vi "Head_Servo_Write.vi"(10 "Stop":bool, 11 "Calibrated Oculus Data":T1) -> ()   [LabVIEW 2017]
uses:
  Calibrated Oculus Data.ctl
  <vilib>/myRIO/Instrument Drivers/Onboard IO/PWM/typedefs/PWM Reference.ctl
  <vilib>/myRIO/Common/Instrument Driver Framework/Utilities/typedefs/myRIO Generic Hardware Reference.ctl
  <vilib>/myRIO/Common/Instrument Driver Framework/Utilities/typedefs/Hardware Version Enum.ctl
  <vilib>/myRIO/Common/Instrument Driver Framework/Utilities/typedefs/myRIO v1.0 Reference.ctl
  <vilib>/myRIO/Common/Instrument Driver Framework/Utilities/typedefs/Generic FPGA Reference.ctl
  <vilib>/myRIO/Common/Instrument Driver Framework/myRIO v1.0/PWM/typedefs/PWM Channels Enum.ctl
  <vilib>/myRIO/Instrument Drivers/Onboard IO/PWM/typedefs/PWM Configuration.ctl
  <vilib>/userdefined/High Color/nirio_resource_hc.ctl
  <vilib>/myRIO/Common/Instrument Driver Framework/Utilities/vis/Is FPGA Ref Available.vi
  <vilib>/myRIO/Common/Instrument Driver Framework/myRIO v1.0/PWM/vis/myRIO v1.1 Open PWM.vi
  <vilib>/myRIO/Instrument Drivers/Onboard IO/PWM/vis/Set Duty Cycle and Frequency.vi
  <vilib>/myRIO/Common/Instrument Driver Framework/Utilities/vis/Validate Channels.vi
  <vilib>/myRIO/Common/Instrument Driver Framework/myRIO v1.0/PWM/vis/myRIO v1.0 Reserve PWM.vi
  <vilib>/myRIO/Common/Instrument Driver Framework/myRIO v1.0/PWM/vis/myRIO v1.0 Build MUX Configuration PWM.vi
  <vilib>/myRIO/Common/Instrument Driver Framework/myRIO v1.0/Resource Manager/vis/myRIO v1.0 Reserve Channel List.vi
  <vilib>/myRIO/Common/Instrument Driver Framework/myRIO v1.0/Resource Manager/vis/myRIO v1.0 Create Configuration List.vi
  <vilib>/myRIO/Common/Instrument Driver Framework/myRIO v1.0/Resource Manager/vis/myRIO v1.0 Reserve Channel.vi
  <vilib>/myRIO/Common/Instrument Driver Framework/myRIO v1.0/Resource Manager/vis/myRIO v1.0 Unreserve Channel.vi
  <vilib>/myRIO/Common/Instrument Driver Framework/myRIO v1.0/Resource Manager/vis/myRIO v1.0 Build Mutex Name.vi
  <vilib>/Utility/VariantDataType/GetNumericInfo.vi
  <vilib>/Utility/error.llb/Error Cluster From Error Code.vi
  <vilib>/myRIO/Common/Instrument Driver Framework/myRIO v1.0/myRIO v1.1 Open.vi
  <vilib>/myRIO/Common/Instrument Driver Framework/Utilities/vis/IO Manager.vi
  <vilib>/myRIO/Common/Instrument Driver Framework/Utilities/vis/Configuration Manager.vi
  <vilib>/myRIO/Common/Instrument Driver Framework/myRIO v1.0/Resource Manager/vis/myRIO v1.0 Configure IO.vi
  <vilib>/myRIO/Common/Instrument Driver Framework/myRIO v1.0/myRIO v1.0 Close.vi
  <vilib>/myRIO/Common/Instrument Driver Framework/myRIO v1.0/PWM/vis/myRIO v1.0 Write PWM.vi
  <vilib>/express/express arith-compare/Formula/XNode/ExpressFormulaBlockNode.xnode
  <vilib>/myRIO/Express VI/Onboard IO/PWM/PWM Express VI.xnode
  <vilib>/myRIO/Instrument Drivers/Onboard IO/PWM/vis/myRIO PWM Open.xnode
  <vilib>/myRIO/Instrument Drivers/Onboard IO/PWM/PWM.lvlib
panel:
  in  "error in":errorcluster
  out "error out":errorcluster
  in  "Pich Offset":dbl
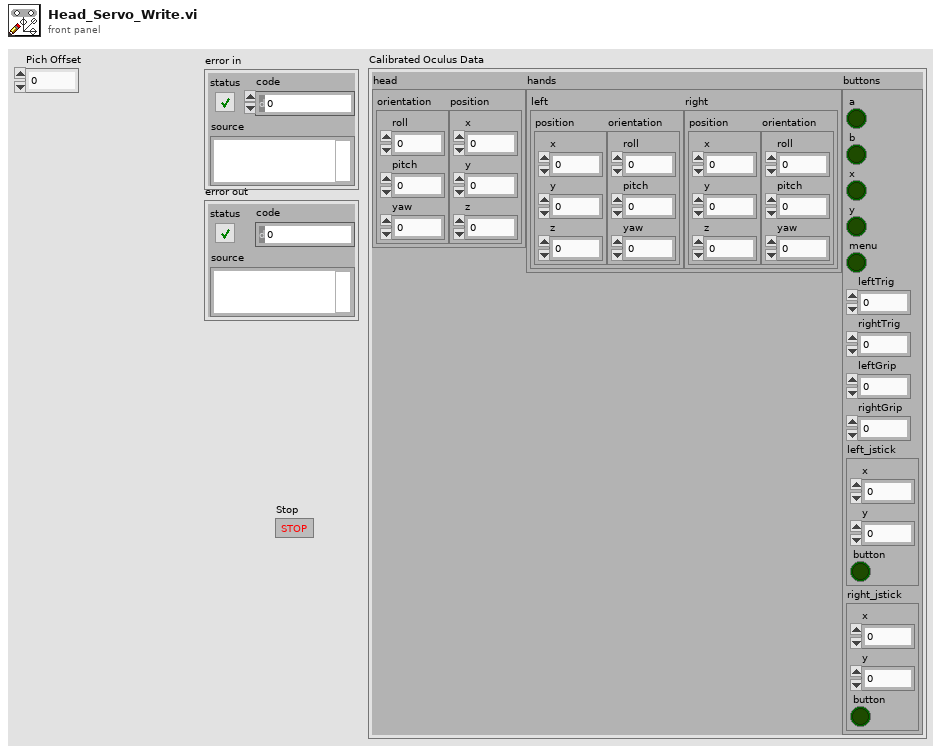
[diagram p1: front panel]
types:
  T1 = typedef "Calibrated Oculus Data.ctl" = cluster{"head":cluster{"orientation":cluster{"roll":dbl, "pitch":dbl, "yaw":dbl}, "position":cluster{"x":dbl, "y":dbl, "z":dbl}}, "hands":cluster{"left":cluster{"position":cluster{"x":dbl, "y":dbl, "z":dbl}, "orientation":cluster{"roll":dbl, "pitch":dbl, "yaw":dbl}}, "right":cluster{"position":cluster{"x":dbl, "y":dbl, "z":dbl}, "orientation":cluster{"roll":dbl, "pitch":dbl, "yaw":dbl}}}, "buttons":cluster{"a":bool, "b":bool, "x":bool, "y":bool, "menu":bool, "leftTrig":dbl, "rightTrig":dbl, "leftGrip":dbl, "rightGrip":dbl, "left_jstick":cluster{"x":dbl, "y":dbl, "button":bool}, "right_jstick":cluster{"x":dbl, "y":dbl, "button":bool}}}
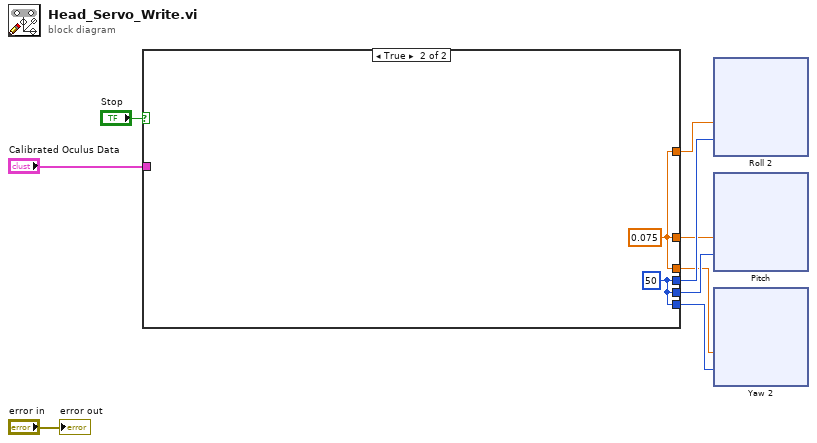
[diagram p0: block diagram]
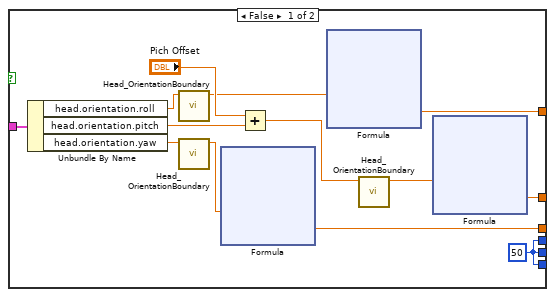
[diagram p2: hidden frame]
diagram:
  n1 = case shown="True" "Stop" {
    tunnel: "Calibrated Oculus Data" -> [w22 _]
    tunnel: [w21 w48] -> w3
    tunnel: [w20 w47] -> w8
    tunnel: [w16 w48] -> w7
    tunnel: [w20 w47] -> w6
    tunnel: [w17 w48] -> w5
    tunnel: [w20 w47] -> w4
    frame False {
      w20 = 50
      n2 = Unbundle By Name(w22) -> ("head.orientation.roll"=w13:dbl, "head.orientation.pitch"=w15:dbl, "head.orientation.yaw"=w19:dbl)
      n3 = call "Head_OrientationBoundary.vi"("Angle in"=w13) -> ("Angle out"=w12:dbl)  [unwired: 10 in]
      n4 = call "Head_OrientationBoundary.vi"("Angle in"=w19) -> ("Angle out"=w18:dbl)  [unwired: 10 in]
      n5 = xnode "Formula"("Angle"=w18) -> ("Result"=w17:dbl)  [unwired: 1 in, 1 out]
      n6 = Add(x="Pich Offset", y=w15) -> (x+y=w11:dbl)
      n7 = xnode "Formula"("Angle"=w12) -> ("Result"=w21:dbl)  [unwired: 1 in, 1 out]
      n8 = call "Head_OrientationBoundary.vi"("Angle in"=w11) -> ("Angle out"=w10:dbl)  [unwired: 10 in]
      n9 = xnode "Formula"("Angle"=w10) -> ("Result"=w16:dbl)  [unwired: 1 in, 1 out]
    }
    frame True {
      w47 = 50
      w48 = 0.075
    }
  }
  n10 = xnode "Roll 2"("Duty Cycle"=w3, "Frequency [Hz]"=w8) -> ()  [unwired: 1 in, 1 out]
  n11 = xnode "Pitch"("Duty Cycle"=w7, "Frequency [Hz]"=w6) -> ()  [unwired: 1 in, 1 out]
  n12 = xnode "Yaw 2"("Duty Cycle"=w5, "Frequency [Hz]"=w4) -> ()  [unwired: 1 in, 1 out]
  "error out" <- "error in"
